vi "dfd_Group Delay_Coefficients Plus.vi"(9 "Gradients":cluster{"r":dbl[], "theta":dbl[], "offset":dbl}, 10 "Coefficients (in)":cluster{"r":dbl[], "theta":dbl[], "offset":dbl}, 11 "Group Delay Design Info":T1={"p"=2, "freq grid"=[], "d"=[], "weight"=[], "Order"=0, "radius"=0.0}) -> (2 "Coefficients (out)":cluster{"r":dbl[], "theta":dbl[], "offset":dbl}, 3 "Group Delay Design Info (dup)":T1={"p"=2, "freq grid"=[], "d"=[], "weight"=[], "Order"=0, "radius"=0.0})   [LabVIEW 2017, in "NI_DigFilter_Design.lvlib"]
uses:
  <vilib>/addons/Digital Filter Design/NI_DigFilter_Design.lvlib
  <vilib>/addons/Digital Filter Design/_GroupDelay.llb/dfd_Group Delay_Design Info.ctl
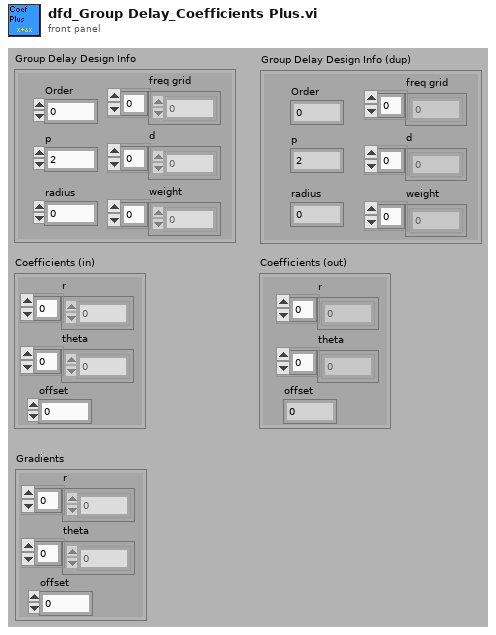
[diagram p1: front panel]
types:
  T1 = typedef "dfd_Group Delay_Design Info.ctl" = cluster{"p":i32, "freq grid":dbl[], "d":dbl[], "weight":dbl[], "Order":i32, "radius":dbl}
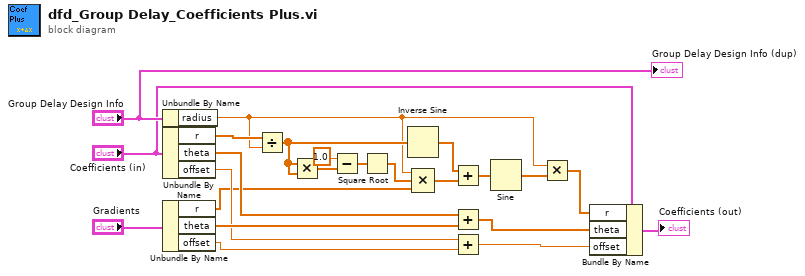
[diagram p0: block diagram]
diagram:
  n1 = Unbundle By Name("Group Delay Design Info") -> ("radius"=w5:dbl)
  n2 = Unbundle By Name("Coefficients (in)") -> ("r"=w8:dbl[], "theta"=w22:dbl[], "offset"=w19:dbl)
  n3 = Unbundle By Name("Gradients") -> ("r"=w11:dbl[], "theta"=w21:dbl[], "offset"=w20:dbl)
  n4 = Divide(x=w8, y=w5) -> (x/y=w7:dbl[])
  n5 = Multiply(x=w7, y=w7) -> (x*y=w14:dbl[])
  n6 = Subtract(x=1.0, y=w14) -> (x-y=w12:dbl[])
  n7 = Square Root(x=w12) -> (sqrt(x)=w10:dbl[])
  n8 = Inverse Sine(1:w7) -> (0:w23:dbl[])
  n9 = Compound Arithmetic op=MULTIPLY(w5, w10, w11) -> (w9:dbl[])
  n10 = Add(x=w23, y=w9) -> (x+y=w18:dbl[])
  n11 = Add(x=w22, y=w21) -> (x+y=w16:dbl[])
  n12 = Add(x=w19, y=w20) -> (x+y=w17:dbl)
  n13 = Sine(x=w18) -> (sin(x)=w15:dbl[])
  n14 = Multiply(x=w5, y=w15) -> (x*y=w6:dbl[])
  n15 = Bundle By Name(cluster="Coefficients (in)", "r"=w6, "theta"=w16, "offset"=w17) -> (→"Coefficients (out)":cluster{"r":dbl[], "theta":dbl[], "offset":dbl})
  "Group Delay Design Info (dup)" <- "Group Delay Design Info"
